vi "三控件移位.vi"(7 "需移动的控件":refnum<vi>, 8 "错误输入（无错误）":errorcluster, 9 "终点控件":refnum<vi>, 10 "中间控件":refnum<vi>, 11 "起始控件":refnum<vi>) -> (0 "错误输出":errorcluster, 1 "终点控件输出":refnum<vi>, 2 "中间控件输出":refnum<vi>, 3 "起始控件输出":refnum<vi>, 4 "移动控件输出":refnum<vi>)   [LabVIEW 8.6, in "窗口操作.lvlib"]
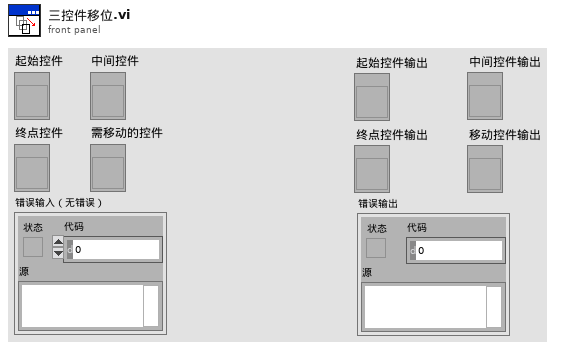
[diagram p1: front panel]
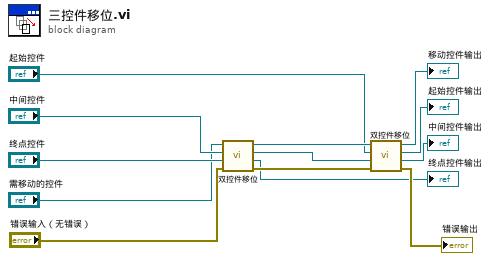
[diagram p0: block diagram]
diagram:
  n1 = call "双控件移位.vi"("错误输入（无错误）"="错误输入（无错误）", "终点控件"="终点控件", "起始控件"="中间控件", "需移动的控件"="需移动的控件") -> ("错误输出"=w13:errorcluster, "终点控件输出"=→"终点控件输出":refnum<vi>, "起始控件输出"=w11:refnum<vi>, "移动控件输出"=w12:refnum<vi>)  [unwired: 4 in]
  n2 = call "双控件移位.vi"("错误输入（无错误）"=w13, "终点控件"=w11, "起始控件"="起始控件", "需移动的控件"=w12) -> ("错误输出"=→"错误输出":errorcluster, "终点控件输出"=→"中间控件输出":refnum<vi>, "起始控件输出"=→"起始控件输出":refnum<vi>, "移动控件输出"=→"移动控件输出":refnum<vi>)  [unwired: 4 in]
